vi "Overflow Magnitude.vi"(6 "Threshold":dbl=1.0, 9 "Input 2":dbl(slide) scale=0.0..10.0, 10 "Input 1":dbl(slide) scale=0.0..10.0) -> (1 "Overflow":bool, 2 "Overflow Magnitude":dbl=1.0)   [LabVIEW 2017]
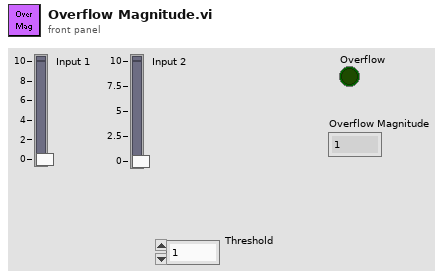
[diagram p1: front panel]
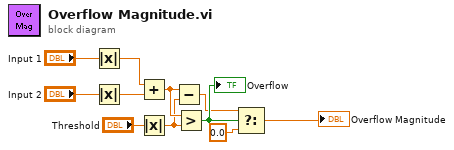
[diagram p0: block diagram]
diagram:
  n1 = Absolute Value(x="Input 1") -> (abs(x)=w8:dbl)
  n2 = Absolute Value(x="Input 2") -> (abs(x)=w10:dbl)
  n3 = Add(x=w8, y=w10) -> (x+y=w5:dbl)
  n4 = Absolute Value(x="Threshold") -> (abs(x)=w4:dbl)
  n5 = Subtract(x=w5, y=w4) -> (x-y=w3:dbl)
  n6 = Greater?(x=w5, y=w4) -> (0:w7:bool)
  "Overflow" <- w7
  n7 = Select(t=w3, s=w7, f=0.0) -> (s? t:f=→"Overflow Magnitude":dbl)
